vi "EXA_getEvent_StateChanged.vi"(8 "error in (no error)":errorcluster, 11 "logevent_StateChanged_Ctl":T1) -> (0 "error out":errorcluster, 2 "function return":i32, 3 "logevent_StateChanged_Ctl out":T1)   [LabVIEW 2016, in "SALLV_EXA.lvlib"]
doc: "int EXA_shm_getEvent_StateChangedLV(EXA_logevent_StateChangedLV *logevent_StateChanged_Ctl );"
uses:
  SALLV_EXA.lvlib
  DataTypes/logevent_StateChanged.ctl
  SALLV_EXA.so
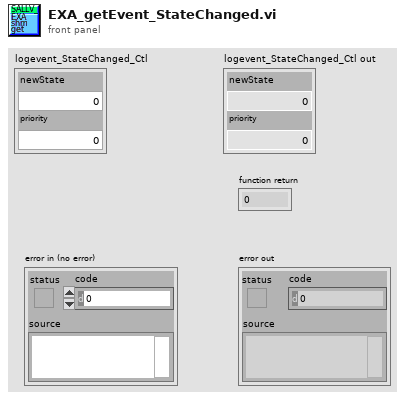
[diagram p1: front panel]
types:
  T1 = typedef "SALLV_EXA.lvlib/logevent_StateChanged.ctl" = cluster{"newState":i32, "priority":i32}
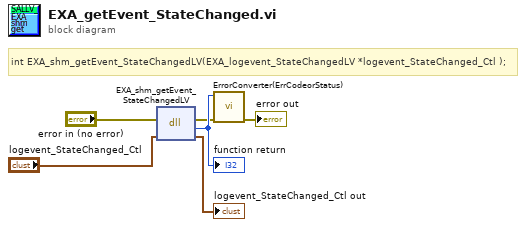
[diagram p0: block diagram]
diagram:
  # "int EXA_shm_getEvent_StateChangedLV(EXA_logevent_StateChangedLV *logevent_StateChanged_Ctl );"
  n1 = dll-call lib="home/andres/Desktop/EXA_SAL_LV/SALLV_EXA.*" fn="EXA_shm_getEvent_StateChangedLV"(error in="error in (no error)", "logevent_StateChanged_Ctl"="logevent_StateChanged_Ctl") -> (error out=w2:errorcluster, w6:i32, "logevent_StateChanged_Ctl"=→"logevent_StateChanged_Ctl out":T1)  [unwired: 2 in, 1 out]
  "function return" <- w6
  n2 = call "ErrorConverter(ErrCodeorStatus).vi"("error in (no error)"=w2, "error code"=w6) -> ("error out"=→"error out":errorcluster)  [unwired: 9 in]
